vi "Configure Offset Angle.vi"(8 "error in (no error)":errorcluster, 10 "ccw offset angle (rad)":dbl, 11 "NI_Robotics_Starter Kit Servo Motor_2.0 in":refnum<class "NI_Robotics_Starter Kit Servo Motor_2.0.lvclass">) -> (0 "error out":errorcluster, 3 "NI_Robotics_Starter Kit Servo Motor_2.0 out":refnum<class "NI_Robotics_Starter Kit Servo Motor_2.0.lvclass">)   [LabVIEW 2017, in "NI_Robotics_Starter Kit Servo Motor_2.0.lvclass"]
uses:
  <vilib>/robotics/Starter Kit/Servo Motor 2.0/NI_Robotics_Starter Kit Servo Motor_2.0.lvclass
  <vilib>/robotics/Starter Kit/Servo Motor 2.0/NI_Robotics_Starter Kit Servo Motor_2.0.lvclass/NI_Robotics_Starter Kit Servo Motor_2.0.ctl
  <instrlib>/Hitec HS400 Series/HAIOL/Hitec HS400 Series.lvclass
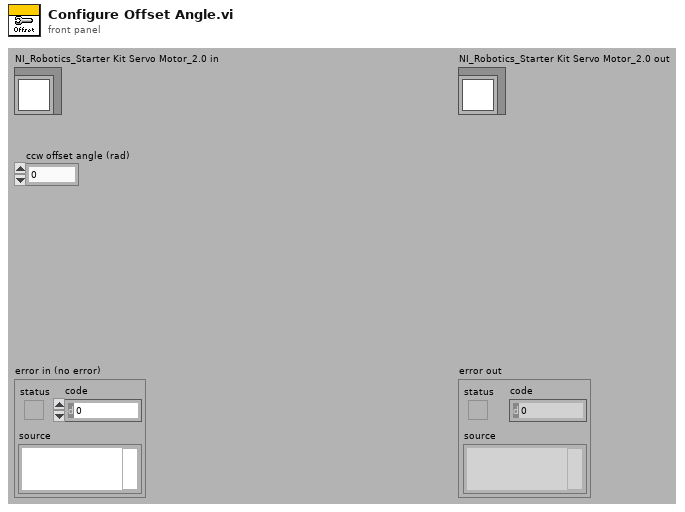
[diagram p1: front panel]
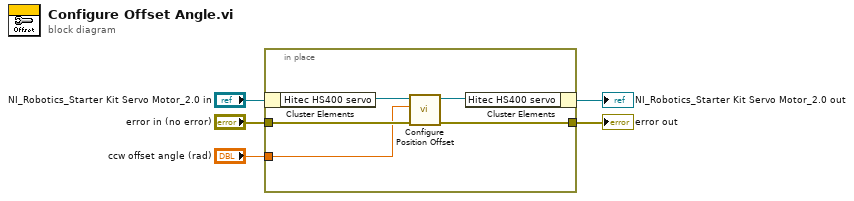
[diagram p0: block diagram]
diagram:
  n1 = in-place {
    in-place-border: "error in (no error)" -> [w8]
    in-place-border: [w7] -> w2
    in-place-border: "ccw offset angle (rad)" -> [w6]
    n2 = in-place-cluster #1("NI_Robotics_Starter Kit Servo Motor_2.0 in") -> ("Hitec HS400 servo"=w10:refnum<class "Hitec HS400 Series.lvclass">)
    n3 = call-dynamic "Configure Position Offset.vi"("error in (no error)"=w8, "CCW Position Offset (0.0 rad)"=w6, "Hitec HS400 Series in"=w10) -> ("error out"=w7:errorcluster, "Hitec HS400 Series out"=w9:refnum<class "Hitec HS400 Series.lvclass">)  [unwired: 7 in]
    n4 = in-place-cluster #1("Hitec HS400 servo"=w9) -> (→"NI_Robotics_Starter Kit Servo Motor_2.0 out":refnum<class "NI_Robotics_Starter Kit Servo Motor_2.0.lvclass">)
  }
  "error out" <- w2
